vi "Gatilho de aquisição em linha.vi"() -> ()   [LabVIEW 2020]
uses:
  <vilib>/vision/Measure.llb/Edge New.ctl
panel:
  out "Salvando peças":bool
  out "Peça detectada":bool
  out "Image":T1(plugin-control)
  out "Edge Information (Edge Detector 1)":T2[](array[typedef]) {"Distance (Real-World)" format="%.2f"; "Location (Real-World)"."Y" format="%.2g"; "Location (Real-World)"."X" format="%.2f"; "Noise" format="%.2f"; "Location (Pixel)"."Y" format="%.2g"; "Location (Pixel)"."X" format="%.2f"; "Strength" format="%.2f"; "Distance (Pixel)" format="%.2f"}
  in  "Stop (F)":bool
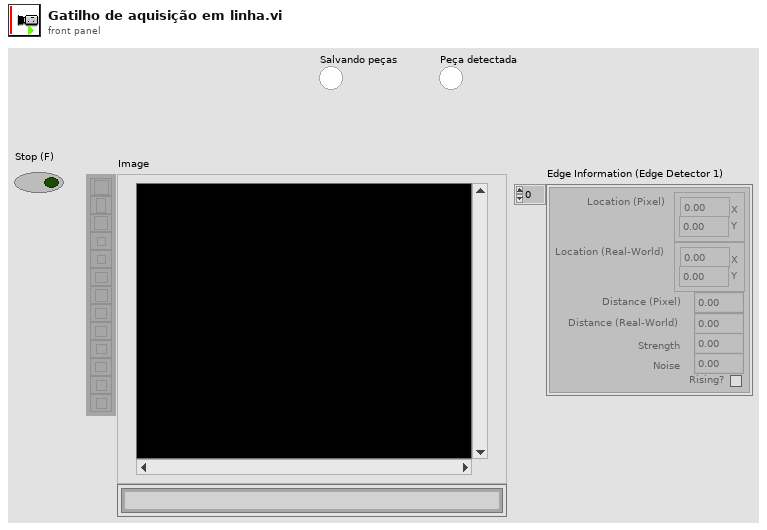
[diagram p1: front panel]
types:
  T1 = typedef "IMAQ Image.ctl" = refnum<image>
  T2 = typedef "Edge New.ctl" = cluster{"Location (Pixel)":cluster{"X":sgl, "Y":sgl}, "Location (Real-World)":cluster{"X":sgl, "Y":sgl}, "Distance (Pixel)":dbl, "Distance (Real-World)":dbl, "Strength":dbl, "Noise":dbl, "Rising?":bool}
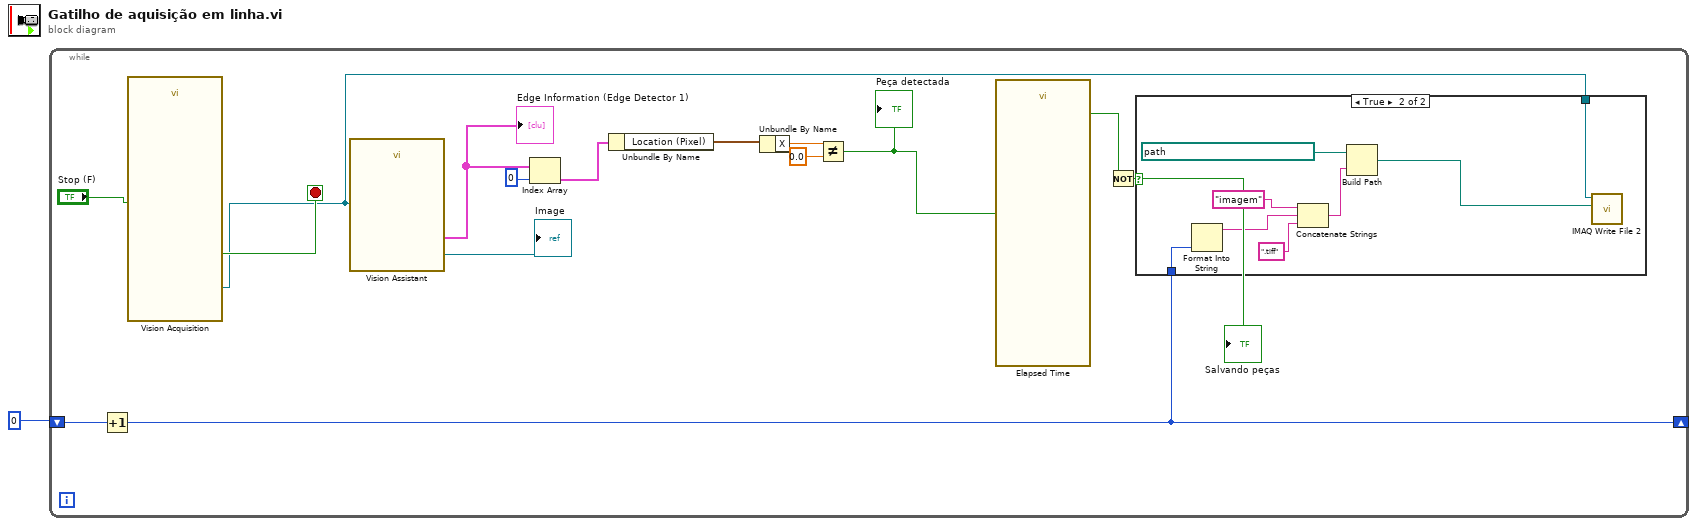
[diagram p0: block diagram]
diagram:
  n1 = while {
    shift-right: [w2] -> _
    shift-left: 0 -> [w3]
    stop <- w15 stop-if-true
    n2 = Increment(x=w3) -> (x+1=w2:i32)
    n3 = call "Vision Acquisition"("Stop (F)"="Stop (F)") -> ("Image Out"=w5:T1, "Stopped"=w15:bool)  [unwired: 22 in, 3 out]
    n4 = call "Vision Assistant"("Image In"=w5) -> ("Image Out"=→"Image":T1, "Edge Information (Edge Detector 1)"=w13:T2[])  [unwired: 24 in, 1 out]
    "Edge Information (Edge Detector 1)" <- w13
    n5 = Index Array(array=w13, index=0) -> (element=w11:T2)
    n6 = Unbundle By Name(w11) -> ("Location (Pixel)"=w10:cluster{"X":sgl, "Y":sgl})
    n7 = Unbundle By Name(w10) -> ("X"=w9:sgl)
    n8 = Not Equal?(x=w9, y=sgl 0.0) -> (x != y?=w7:bool)
    "Peça detectada" <- w7
    n9 = call "Elapsed Time"("Reset"=w7) -> ("Time has Elapsed"=w6:bool)  [unwired: 11 in, 7 out]
    n10 = Not(x=w6) -> (.not. x?=w4:bool)
    "Salvando peças" <- w4
    n11 = case shown="True" w4 {
      tunnel: w5 -> [_ w24]
      tunnel: w2 -> [_ w21]
      frame False {
      }
      frame True {
        n12 = Format Into String(w21) -> (resulting string=w20:string)  [unwired: 3 in, 1 out]
        n13 = Concatenate Strings("imagem" ("string"), w20, ".tiff" ("string")) -> (w18:string)
        n14 = Build Path(base path=path "C:/Users/Beneli/Desktop/peça", name or relative path=w18) -> (appended path=w17:path)
        n15 = call-poly "IMAQ Write File 2"("File Path"=w17, "Image"=w24) -> ()  [unwired: 8 in, 2 out]
      }
    }
  }
